vi "Usage Statistics.vi"(11 "Operation":enum16{"Increment Read", "Increment Write"}(ring)) -> ()   [LabVIEW 2017]
uses:
  <vilib>/Rock Robotics/Network Tables/NT Globals.vi
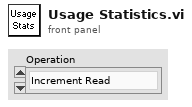
[diagram p1: front panel]
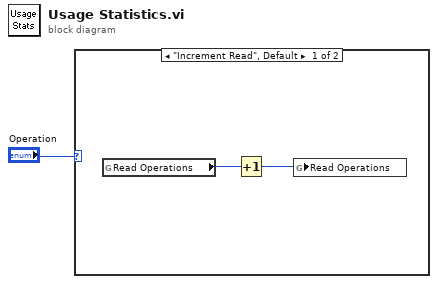
[diagram p0: block diagram]
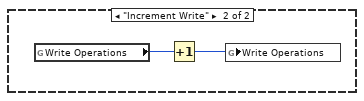
[diagram p2: hidden frame]
diagram:
  n1 = case shown="\"Increment Read\", Default" "Operation" {
    frame "Increment Read", Default {
      n2 = global read "NT Globals.vi" "Read Operations"() -> (w3:i32)
      n3 = Increment(x=w3) -> (x+1=w2:i32)
      n4 = global write "NT Globals.vi" "Read Operations"(w2) -> ()
    }
    frame "Increment Write" {
      n5 = global read "NT Globals.vi" "Write Operations"() -> (w5:i32)
      n6 = Increment(x=w5) -> (x+1=w4:i32)
      n7 = global write "NT Globals.vi" "Write Operations"(w4) -> ()
    }
  }
